vi "Is OS 64 Bit.vi"(8 "error in (no error)":errorcluster, 11 "Detection Method":T1(ring)) -> (0 "error out":errorcluster, 3 "Is 64 Bit OS?":bool)   [LabVIEW 2019, in "Tools.lvlib"]
uses:
  <vilib>/registry/registry.llb/Registry SAM.ctl
  Tools.lvlib
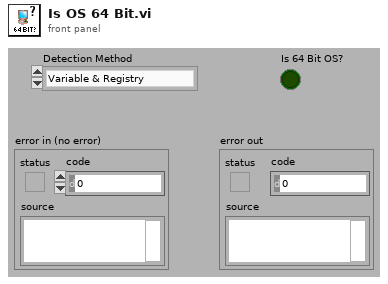
[diagram p1: front panel]
types:
  T1 = enum16{"Variable & Registry", "Variable", "Registry"}
  T2 = typedef "Registry SAM.ctl" = enum32{"KEY_QUERY_VALUE", "KEY_SET_VALUE", "KEY_CREATE_SUB_KEY", "KEY_ENUMERATE_SUB_KEYS", "KEY_NOTIFY", "KEY_CREATE_LINK", "KEY_READ", "KEY_WRITE", "KEY_ALL_ACCESS", "KEY_READ | KEY_WRITE"}
  T3 = typedef "Registry refnum.ctl" = refnum<k1>
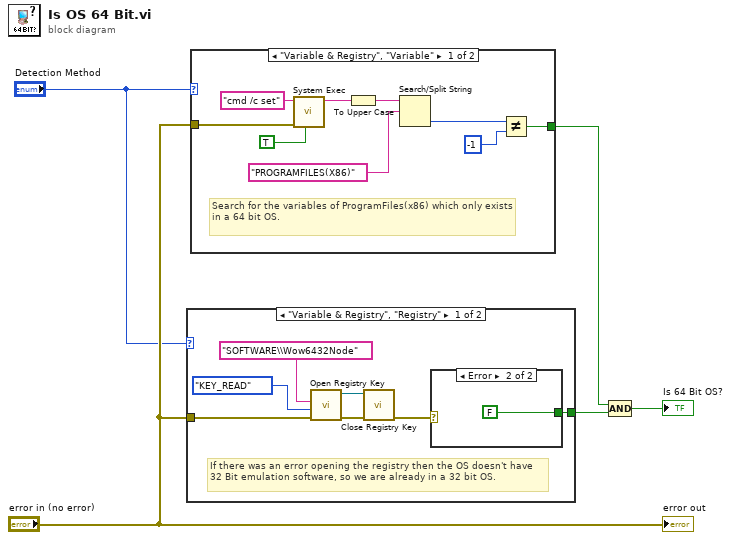
[diagram p0: block diagram]
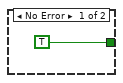
[diagram p2: hidden frame]
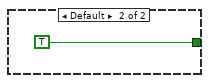
[diagram p3: hidden frame]
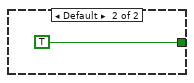
[diagram p4: hidden frame]
diagram:
  n1 = case shown="\"Variable & Registry\", \"Registry\"" "Detection Method" {
    tunnel: "error in (no error)" -> [w7 _]
    tunnel: [w6 TRUE] -> w4
    frame "Variable & Registry", "Registry" {
      # "If there was an error opening the registry then the OS doesn't have 32 Bit emulation software, so we are already in a 32 bit OS."
      n2 = call <vilib>:"Open Registry Key.vi"("error in (no error)"=w7, "security access mask (KEY_READ | KEY_WRITE)"=Registry_SAM."KEY_READ", "subkey"="SOFTWARE\\Wow6432Node") -> ("error out"=w11:errorcluster, "refnum out"=w10:T3)  [unwired: 7 in]
      n3 = call <vilib>:"Close Registry Key.vi"("error in (no error)"=w11, "refnum"=w10) -> ("error out"=w8:errorcluster)  [unwired: 5 in]
      n4 = case shown="Error" w8 {
        tunnel: [TRUE FALSE] -> w6
        frame No Error {
        }
        frame Error {
        }
      }
    }
    frame Default {
    }
  }
  n5 = case shown="\"Variable & Registry\", \"Variable\"" "Detection Method" {
    tunnel: "error in (no error)" -> [w24 _]
    tunnel: [w16 TRUE] -> w3
    frame "Variable & Registry", "Variable" {
      # "Search for the variables of ProgramFiles(x86) which only exists in a 64 bit OS."
      n6 = call <vilib>:"System Exec.vi"("run minimized? (F)"=TRUE, "error in (no error)"=w24, "command line"="cmd /c set") -> ("standard output"=w21:string)  [unwired: 5 in, 3 out]
      n7 = To Upper Case(1:w21) -> (0:w20:string)
      n8 = Search/Split String(string=w20, search string/char (-)="PROGRAMFILES(X86)") -> (offset of match=w18:i32)  [unwired: 1 in, 2 out]
      n9 = Not Equal?(x=w18, y=-1) -> (x != y?=w16:bool)
    }
    frame Default {
    }
  }
  n10 = Compound Arithmetic op=AND(w3, w4) -> (→"Is 64 Bit OS?":bool)
  "error out" <- "error in (no error)"
